vi "~_niRFUtil FTW VBW Filter (IIR).vi"(0 "Waveform In":T1 {"y" min=0 max=127 format="%.2f"; "dx" format="%^.2e"; "x0" format="%^.2e"}, 2 "Initial Condition":dbl, 5 "VBW (Hz)":dbl format="%.3p") -> (4 "Waveform Out":T1 {"y" min=0 max=127 format="%.2f"; "dx" format="%^.2e"; "x0" format="%^.2e"})   [LabVIEW 2016]
uses:
  niRFUtil/Includes/niRFUtil INC Real Waveform.ctl
  niRFUtil/Includes/niRFUtil INC Real Array.ctl
  niRFUtil/niRFUtil.lvlib
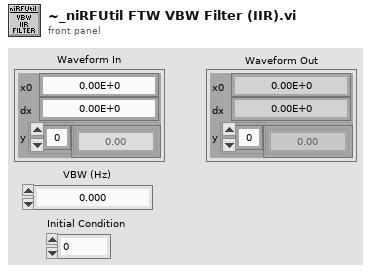
[diagram p1: front panel]
types:
  T1 = typedef "niRFUtil.lvlib/niRFUtil INC Real Waveform.ctl" = cluster{"x0":dbl, "dx":dbl, "y":T2}
  T2 = typedef "niRFUtil.lvlib/niRFUtil INC Real Array.ctl" = sgl[]
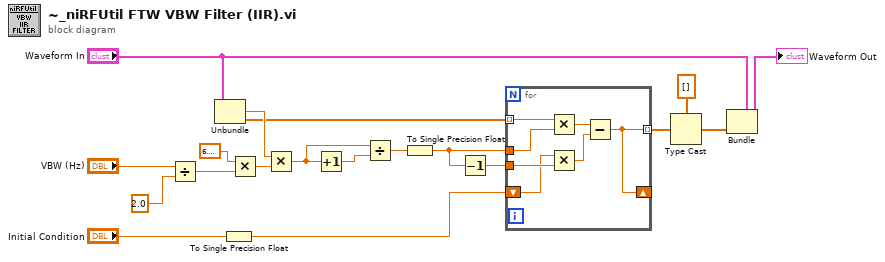
[diagram p0: block diagram]
diagram:
  n1 = Divide(x="VBW (Hz)", y=2.0) -> (x/y=w17:dbl)
  n2 = Unbundle("Waveform In") -> ("dx"=w12:dbl, "y"=w5:T2)  [unwired: 1 out]
  n3 = To Single Precision Float(number="Initial Condition") -> (single precision float=w7:sgl)
  n4 = Multiply(x=6.283185307179586, y=w17) -> (x*y=w15:dbl)
  n5 = Multiply(x=w12, y=w15) -> (x*y=w13:dbl)
  n6 = Increment(x=w13) -> (x+1=w14:dbl)
  n7 = Divide(x=w13, y=w14) -> (x/y=w10:dbl)
  n8 = To Single Precision Float(number=w10) -> (single precision float=w8:sgl)
  n9 = Decrement(x=w8) -> (x-1=w11:sgl)
  n10 = for {
    tunnel: w5 -> [w26] mode=indexing
    tunnel: w8 -> [w25]
    tunnel: w11 -> [w24]
    tunnel: [w21] -> w3 mode=indexing
    shift-right: [w21] -> _
    shift-left: w7 -> [w20]
    n11 = Multiply(x=w26, y=w25) -> (x*y=w23:sgl)
    n12 = Multiply(x=w20, y=w24) -> (x*y=w22:sgl)
    n13 = Subtract(x=w23, y=w22) -> (x-y=w21:sgl)
  }
  n14 = Type Cast(type=T2 [] ("y"), x=w3) -> (*(type *) &x=w1:T2)
  n15 = Bundle(cluster="Waveform In", "y"=w1) -> (→"Waveform Out":T1)  [unwired: 2 in]
